vi "Test INFO-Logger.vi"(8 "error in":errorcluster) -> (0 "error out":errorcluster)   [LabVIEW 2016, in "UT_Helper.lvlib"]
doc: "Test correct function of the Info-Logger."
uses:
  UT_Helper.lvlib
  Source/HSE-Logger/LogLevel.ctl
  Source/HSE-Logger/LogRecord/LogRecord.lvclass/LogRecord.ctl
  Source/HSE-Logger/LogRecord/Get Level.vi
  Source/HSE-Logger/LogRecord/Get Message.vi
  Source/HSE-Logger/LogRecord/Get Error.vi
  Source/HSE-Logger/Handler/UserEventHandler/UserEventHandler.lvclass
  C:/Users/admin/_Git/hse-logger/Source/HSE-Logger/Handler/Handler.lvclass
  <vilib>/addons/_JKI Toolkits/Caraya/classes/Test/Test.lvclass
  Source/HSE-Logger/hse-logger.lvlib
  <vilib>/addons/_JKI Toolkits/Caraya/classes/Assert/Assert.lvclass
  Source/HSE-Logger/LogRecord/LogRecord.lvclass
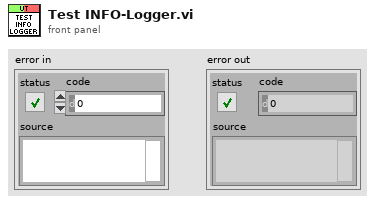
[diagram p1: front panel]
types:
  T1 = typedef "hse-logger.lvlib/LogLevel.ctl" = enum16{"DEBUG", "INFO", "WARNING", "ERROR", "CRITICAL"}
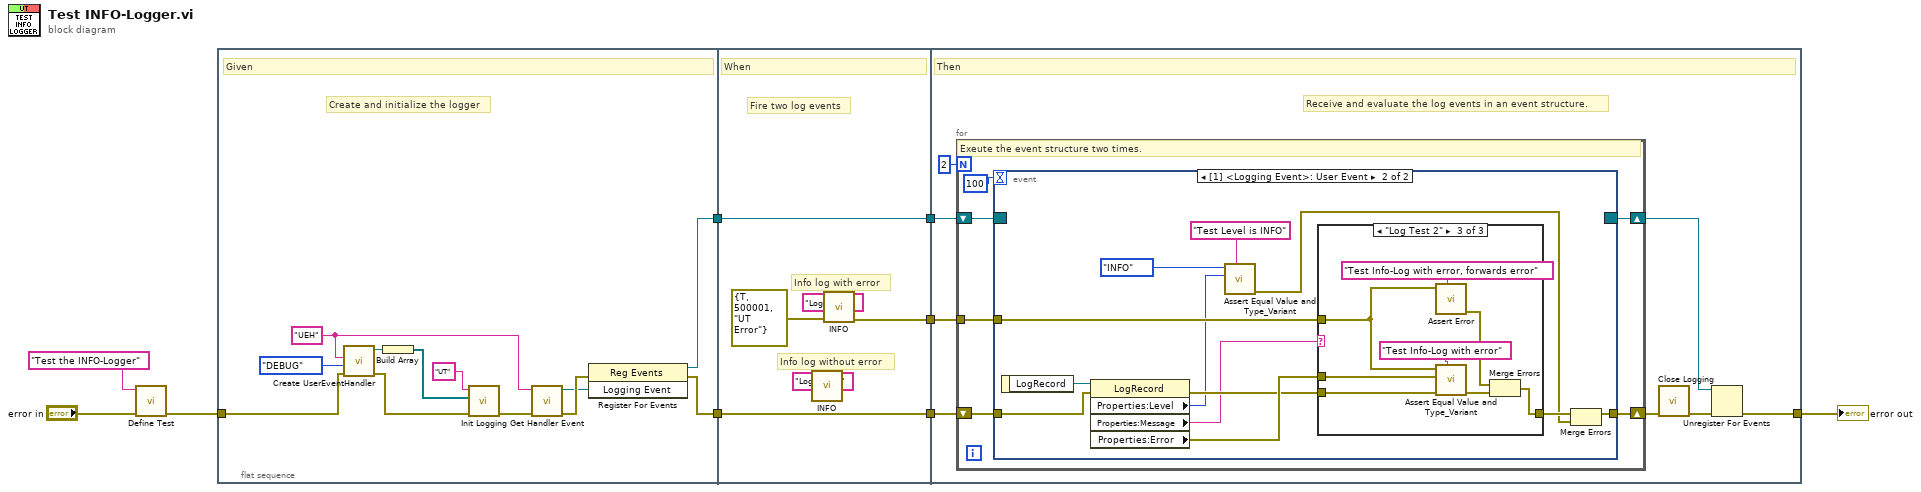
[diagram p0: block diagram]
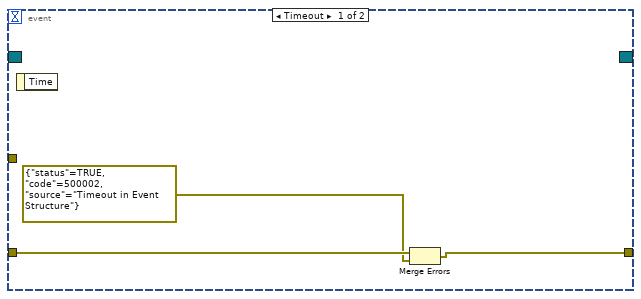
[diagram p2: hidden frame]
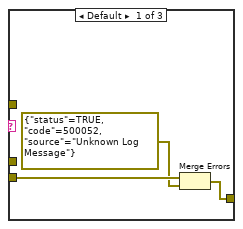
[diagram p3: hidden frame]
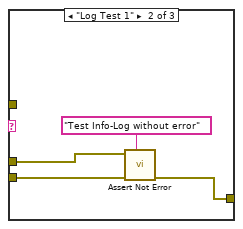
[diagram p4: hidden frame]
diagram:
  n1 = call <vilib>:"Define Test.vi"("error in (no error)"="error in", "Label (VI Title)"="Test the INFO-Logger") -> ("error out"=w6:errorcluster)  [unwired: 8 in, 1 out]
  n2 = flat-sequence {
    tunnel: w6 -> [w20]
    tunnel: [w17] -> w9
    tunnel: [w12] -> w2
    tunnel: w9 -> [w27]
    tunnel: [w27] -> w5
    tunnel: w2 -> [w23]
    tunnel: [w23] -> w1
    tunnel: [w25] -> w4
    tunnel: [w31] -> w8
    tunnel: w5 -> [w35]
    tunnel: w1 -> [w30]
    tunnel: w4 -> [w34]
    frame #0 {
      w11 = "UEH" ("Name")
      # "Create and initialize the logger"
      # "Given"
      n3 = call "Create UserEventHandler.vi"("error in"=w20, "Level"=LogLevel."DEBUG", "Name"=w11) -> ("error out"=w19:errorcluster, "UserEventHandler out"=w16:refnum<class "UserEventHandler.lvclass">)  [unwired: 7 in]
      n4 = Build Array(w16) -> (w15:refnum<class "UserEventHandler.lvclass">[])
      n5 = call "Init Logging.vi"("error in"=w19, "Handlers"=w15, "Name"="UT") -> ("error out"=w18:errorcluster)  [unwired: 8 in]
      n6 = call "Get Handler Event.vi"("error in"=w18, "Name"=w11) -> ("error out"=w21:errorcluster, "Logging Event"=w13:refnum<user-event>)  [unwired: 8 in]
      n7 = register-events(error in=w21, w13) -> (reference out=w12:refnum<event-registration>, error out=w17:errorcluster)  [unwired: 1 in]
    }
    frame #1 {
      # "Info log with error"
      # "Info log without error"
      # "Fire two log events"
      # "When"
      n8 = call "INFO.vi"("Message"="Log Test 1") -> ()  [unwired: 10 in, 1 out]
      n9 = call "INFO.vi"("Message"="Log Test 2", "error in"=errorcluster {"status"=TRUE, "code"=500001, "source"="UT Error"}) -> ("error out"=w25:errorcluster)  [unwired: 9 in]
    }
    frame #2 {
      # "Receive and evaluate the log events in an event structure."
      # "Then"
      n10 = for {
        N: 2 -> [_]
        shift-right: [w40] -> w33
        shift-left: w35 -> [w41]
        tunnel: w34 -> [w39]
        shift-right: [w36] -> w28
        shift-left: w30 -> [w38]
        # "Exeute the event structure two times."
        n11 = event shown="[1] <Logging Event>: User Event" {
          selector: w38 -> [_ _]
          dyn-events: [_ _] -> w36
          timeout: 100 -> [_ _]
          tunnel: w41 -> [w44 w51]
          tunnel: [w42 w54] -> w40
          tunnel: w39 -> [_ w55]
          event Timeout {
            n12 = event-data() -> ()  [unwired: 1 in, 1 out]
            n13 = Merge Errors(w44, errorcluster {"status"=TRUE, "code"=500002, "source"="Timeout in Event Structure"} ("error out")) -> (w42:errorcluster)
          }
          event User Event {
            n14 = event-data() -> ("LogRecord"=w47:refnum<class "LogRecord.lvclass">)  [unwired: 1 in]
            n15 = property class="LogRecord"(reference=w47, error in=w51) -> (error out=w50:errorcluster, "Properties:Level"=w46:T1, "Properties:Message"=w45:string, "Properties:Error"=w52:errorcluster)  [unwired: 1 out]
            n16 = call <vilib>:"Assert Equal Value and Type_Variant.vi"("Label"="Test Level is INFO", "Y"=w46, "X"=LogLevel."INFO" ("Level")) -> ("error out"=w53:errorcluster)  [unwired: 7 in, 1 out]
            n17 = case shown="\"Log Test 2\"" w45 {
              tunnel: w52 -> [_ w62 w69]
              tunnel: w50 -> [w59 w63 w71]
              tunnel: [w57 w61 w67] -> w56
              tunnel: w55 -> [_ _ w68]
              frame Default {
                n18 = Merge Errors(w59, errorcluster {"status"=TRUE, "code"=500052, "source"="Unknown Log Message"} ("error out")) -> (w57:errorcluster)
              }
              frame "Log Test 1" {
                n19 = call <vilib>:"Assert Not Error.vi"("Label"="Test Info-Log without error", "error in (no error)"=w63, "Not Error?"=w62) -> ("error out"=w61:errorcluster)  [unwired: 7 in, 1 out]
              }
              frame "Log Test 2" {
                n20 = call <vilib>:"Assert Error.vi"("Label"="Test Info-Log with error, forwards error", "Error?"=w68) -> ("error out"=w66:errorcluster)  [unwired: 8 in, 1 out]
                n21 = call <vilib>:"Assert Equal Value and Type_Variant.vi"("Label"="Test Info-Log with error", "error in (no error)"=w71, "Y"=w69, "X"=w68) -> ("error out"=w70:errorcluster)  [unwired: 6 in, 1 out]
                n22 = Merge Errors(w66, w70) -> (w67:errorcluster)
              }
            }
            n23 = Merge Errors(w56, w53) -> (w54:errorcluster)
          }
        }
      }
      n24 = call "Close Logging.vi"("error in"=w33) -> ("error out"=w32:errorcluster)  [unwired: 10 in]
      n25 = Unregister For Events(event registration refnum=w28, error in=w32) -> (error out=w31:errorcluster)
    }
  }
  "error out" <- w8
